vi "CubicSplineInterpolating.vi"() -> ()   [LabVIEW 2016]
uses:
  <vilib>/Analysis/baseanly.llb/Real Inverse Matrix.vi
  <vilib>/Analysis/Matrix/Numeric/Multiply/Multiply - RM,RM.vi
  <vilib>/Analysis/polynomials.llb/Polynomial Plot (Range).vi
  <vilib>/Analysis/NI_AALBase.lvlib
  <vilib>/Analysis/Matrix/NI_Matrix.lvlib
  <vilib>/Analysis/NI_AALPro.lvlib
panel:
  out "XY Graph":cluster{dbl[], "P(A)":dbl[]}(graph)
  in  "End Angle":dbl
  in  "Start Angle":dbl
  in  "Waypoints":dbl[][](array[numeric])
  # "in degrees"
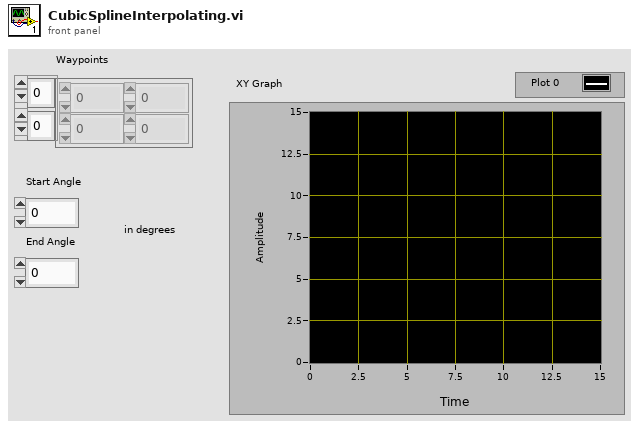
[diagram p1: front panel]
types:
  T1 = typedef "NI_Matrix.lvlib/RealMatrix.ctl" = dbl[][]
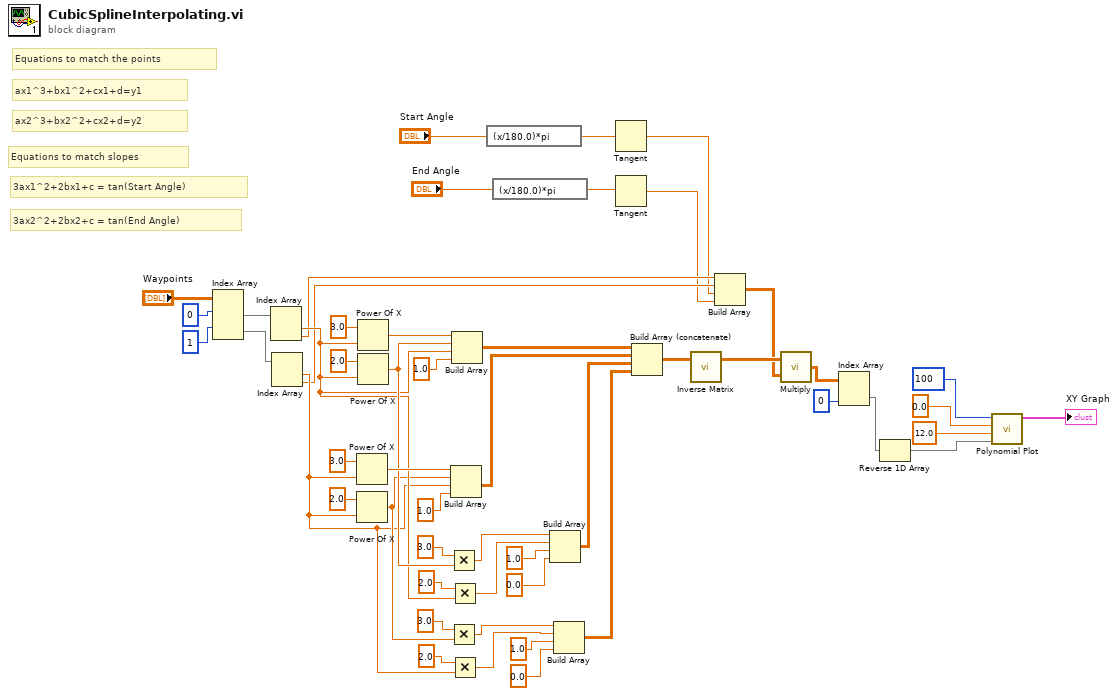
[diagram p0: block diagram]
diagram:
  # "Equations to match slopes"
  # "3ax2^2+2bx2+c = tan(End Angle)"
  # "3ax1^2+2bx1+c = tan(Start Angle)"
  # "Equations to match the points"
  # "ax2^3+bx2^2+cx2+d=y2"
  # "ax1^3+bx1^2+cx1+d=y1"
  n1 = Index Array(array="Waypoints", index (row) #1=0 ("disabled index (col)"), index (row) #2=1 ("disabled index (col)")) -> (element #1=w49:dbl[], element #2=w48:dbl[])  [unwired: 2 in]
  n2 = Index Array(array=w49) -> (element #1=w27:dbl, element #2=w15:dbl)  [unwired: 2 in]
  n3 = Index Array(array=w48) -> (element #1=w18:dbl, element #2=w14:dbl)  [unwired: 2 in]
  n4 = Power Of X(1:w18, 2:3.0 ("x")) -> (0:w42:dbl)
  n5 = Power Of X(1:w18, 2:2.0 ("x")) -> (0:w19:dbl)
  n6 = Power Of X(1:w27, 2:3.0 ("x")) -> (0:w47:dbl)
  n7 = Power Of X(1:w27, 2:2.0 ("x")) -> (0:w28:dbl)
  n8 = Multiply(x=3.0, y=w28) -> (x*y=w25:dbl)
  n9 = Multiply(x=3.0, y=w19) -> (x*y=w17:dbl)
  n10 = Multiply(x=2.0, y=w27) -> (x*y=w24:dbl)
  n11 = Multiply(x=2.0, y=w18) -> (x*y=w16:dbl)
  n12 = Build Array(w42, w19, w18, 1.0 ("x")) -> (w40:T1)
  n13 = Build Array(w47, w28, w27, 1.0 ("x")) -> (w41:T1)
  n14 = expression code="(x/180.0)*pi" ("degrees to radians")("Start Angle") -> (w36:dbl)
  n15 = expression code="(x/180.0)*pi" ("degrees to radians")("End Angle") -> (w37:dbl)
  n16 = Build Array(w25, w24, 1.0 ("x"), 0.0 ("x")) -> (w23:T1)
  n17 = Build Array(w17, w16, 1.0 ("x"), 0.0 ("x")) -> (w22:T1)
  n18 = Tangent(1:w36) -> (0:w13:dbl)
  n19 = Tangent(1:w37) -> (0:w12:dbl)
  n20 = Build Array (concatenate)(w41, w40, w23, w22) -> (w11:T1)
  n21 = call-poly <vilib>:"Inverse Matrix.vi"("Input Matrix"=w11) -> ("Inverse Matrix"=w10:T1)  [unwired: 1 in, 1 out]
  n22 = Build Array(w15, w14, w13, w12) -> (w9:T1)
  n23 = call-poly <vilib>:"Multiply.vi"("Real Matrix B"=w9, "Real Matrix A"=w10) -> ("A * B"=w8:T1)
  n24 = Index Array(array=w8, index (col)=0 ("disabled index (col)")) -> (element=w2:dbl[])  [unwired: 1 in]
  n25 = Reverse 1D Array(array=w2) -> (reversed array=w1:dbl[])
  n26 = call-poly <vilib>:"Polynomial Plot.vi"("P(x)"=w1, "end"=12.0, "start"=0.0, "samples"=100) -> ("polynomial plot"=→"XY Graph":cluster{"Ramp Pattern":dbl[], "P(A)":dbl[]})  [unwired: 6 in, 1 out]
